vi "CAEN_HVBoard.contents.vi"   [LabVIEW 2014, in "CAEN_HVBoard.lvlib"]
uses:
  CAEN_HVBoard.lvlib
panel:
  # "Refer to blockdiagram for content VIs."
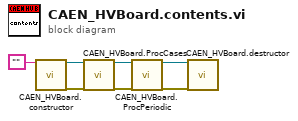
[diagram p0: block diagram]
diagram:
  n1 = call "CAEN_HVBoard.constructor.vi"("name"="") -> ("i ref out"=w3:refnum<vi>, "error out"=w2:errorcluster)  [unwired: 16 in, 1 out]
  n2 = call "CAEN_HVBoard.ProcCases.vi"("i ref in"=w3, "error in (no error)"=w2) -> ("i ref out"=w4:refnum<vi>, "error out"=w5:errorcluster)  [unwired: 15 in, 1 out]
  n3 = call "CAEN_HVBoard.ProcPeriodic.vi"("i ref in"=w4, "error in (no error)"=w5) -> ("i ref out"=w7:refnum<vi>, "error out"=w6:errorcluster)  [unwired: 15 in, 1 out]
  n4 = call "CAEN_HVBoard.destructor.vi"("i ref in"=w7, "error in(no error)"=w6) -> ()  [unwired: 17 in, 1 out]
